vi "CanChannelClose.vi"(3 "error in":errorcluster {"code" format="%.0x"}, 5 "CAN Channel Handle":u32) -> (0 "error out":errorcluster {"code" format="%.0x"})   [LabVIEW 2012]
doc: "Closes the CAN channel specified by the CAN channel handle."
uses:
  vcilva.dll
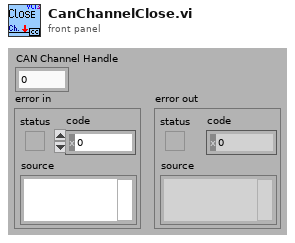
[diagram p1: front panel]
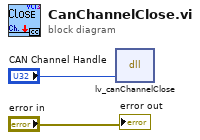
[diagram p0: block diagram]
diagram:
  n1 = dll-call lib="vcilva.dll" fn="lv_canChannelClose"("hCanChn"="CAN Channel Handle") -> ()  [unwired: 5 in, 2 out]
  "error out" <- "error in"
